vi "_Get Row in Worksheet.vi"(8 "error in":errorcluster, 10 "RowIndex":i32, 11 "Worksheet in":refnum<k24>) -> (0 "error out":errorcluster, 2 "Row out":refnum<k24>, 3 "Worksheet out":refnum<k24>)   [LabVIEW 2021, in "Open Xml.lvlib"]
uses:
  Open Xml.lvlib
  D:/git/Open-Xml-LabVIEW/dll/DocumentFormat.OpenXml.dll
  dll/DocumentFormat.OpenXml.dll
  D:/git/Open-Xml-LabVIEW/dll/DocumentFormat.OpenXml.Framework.dll
  dll/DocumentFormat.OpenXml.Framework.dll
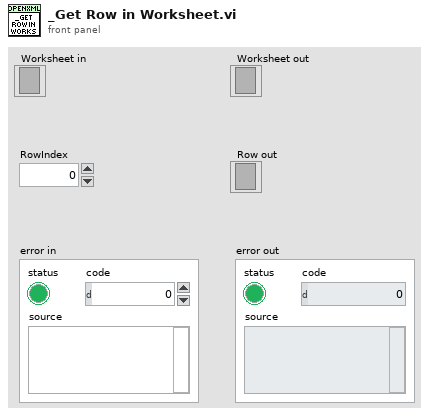
[diagram p1: front panel]
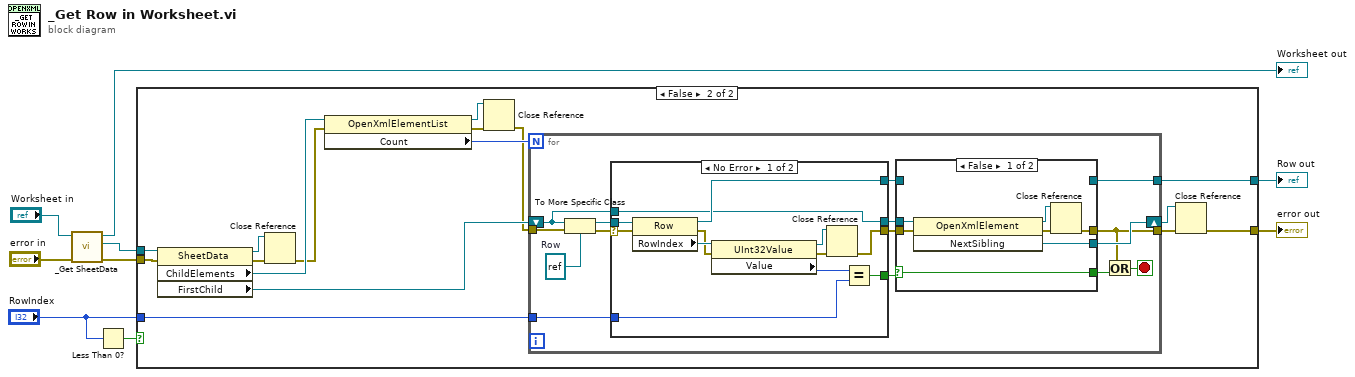
[diagram p0: block diagram]
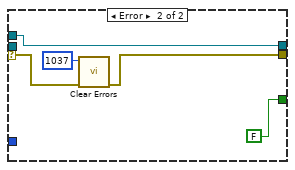
[diagram p3: hidden frame]
diagram:
  n1 = call "_Get SheetData.vi"("error in"="error in", "Worksheet in"="Worksheet in") -> ("error out"=w3:errorcluster, "SheetData"=w2:refnum<k24>, "Worksheet out"=→"Worksheet out":refnum<k24>)  [unwired: 7 in]
  n2 = Less Than 0?(x="RowIndex") -> (x < 0?=w9:bool)
  n3 = case shown="False" w9 {
    tunnel: w2 -> [_ w26]
    tunnel: w3 -> [w10 w23]
    tunnel: [_ w20] -> w6
    tunnel: [w10 w12] -> w7
    tunnel: "RowIndex" -> [_ w21]
    frame True {
    }
    frame False {
      n4 = property class="SheetData"(reference=w26, error in=w23) -> (reference out=w14:refnum<k24>, error out=w18:errorcluster, "ChildElements"=w25:refnum<k24>, "FirstChild"=w22:refnum<k24>)
      n5 = Close Reference(reference=w14, error in (no error)=w18) -> (error out=w15:errorcluster)
      n6 = property class="OpenXmlElementList"(reference=w25, error in=w15) -> (reference out=w19:refnum<k24>, error out=w17:errorcluster, "Count"=w24:i32)
      n7 = Close Reference(reference=w19, error in (no error)=w17) -> (error out=w16:errorcluster)
      n8 = for {
        N: w24 -> [_]
        tunnel: w16 -> [w40]
        tunnel: [w31] -> w13
        shift-right: [w32] -> w11
        shift-left: w22 -> [w38]
        tunnel: w21 -> [w36]
        tunnel: [w28] -> w20
        stop <- w35 stop-if-true
        w41 = refnum<k24> refnum  # Row
        n9 = To More Specific Class(target class=w41, reference=w38, error in=w40) -> (specific class reference=w37:refnum<k24>, error out=w39:errorcluster)
        n10 = case shown="No Error" w39 {
          selector: w39 -> [w53 w58]
          tunnel: [w43 w56] -> w34
          tunnel: w38 -> [w42 w54]
          tunnel: [w42 w54] -> w33
          tunnel: [w48 FALSE] -> w27
          tunnel: w37 -> [w52 _]
          tunnel: w36 -> [w49 _]
          tunnel: [w47 _] -> w29
          frame No Error {
            n11 = property class="Row"(reference=w52, error in=w53) -> (reference out=w47:refnum<k24>, error out=w46:errorcluster, "RowIndex"=w51:refnum<k24>)
            n12 = property class="UInt32Value"(reference=w51, error in=w46) -> (reference out=w44:refnum<k24>, error out=w45:errorcluster, "Value"=w50:u32)
            n13 = Close Reference(reference=w44, error in (no error)=w45) -> (error out=w43:errorcluster)
            n14 = Equal?(x=w50, y=w49) -> (x = y?=w48:bool)
          }
          frame Error {
            n15 = call <vilib>:"Clear Errors.vi"("error in (no error)"=w58, "specific error code to clear (0: all)"=1037) -> ("error out"=w56:errorcluster)  [unwired: 4 in, 1 out]
          }
        }
        n16 = case shown="False" w27 {
          selector: w27 -> [w59 w67]
          tunnel: w34 -> [w65 w68]
          tunnel: w33 -> [w64 _]
          tunnel: [w62 _] -> w32
          tunnel: [w60 w68] -> w31
          tunnel: [w59 w67] -> w30
          tunnel: w29 -> [_ w66]
          tunnel: [_ w66] -> w28
          frame False {
            n17 = invoke class="OpenXmlElement" method="NextSibling"(reference=w64, error in=w65) -> (reference out=w63:refnum<k24>, error out=w61:errorcluster, "NextSibling"=w62:refnum<k24>)  [unwired: 1 in]
            n18 = Close Reference(reference=w63, error in (no error)=w61) -> (error out=w60:errorcluster)
          }
          frame True {
          }
        }
        n19 = Or(x=w31, y=w30) -> (x .or. y?=w35:bool)
      }
      n20 = Close Reference(reference=w11, error in (no error)=w13) -> (error out=w12:errorcluster)
    }
  }
  "error out" <- w7
  "Row out" <- w6
